vi "3-Midbrain.vi"() -> ()   [LabVIEW 2010]
doc: "This VI acts as the MIDbrain in the Olin Robotics Architecture. It interacts with neural clusters on both the Forebrain and Hindbrain as shown in teh respective control panel dynamic documentation diagrams."
uses:
  3-Midbrain/3.3-What/_typedefs/3.3-What Sensor Typedef.ctl
  3-Midbrain/3.3-What/_typedefs/3.3.1-LIDAR Data Typedef.ctl
  4-High Neurons/4.2-Where Sensor Typedef.ctl
  4-High Neurons/Current GPS Data.ctl
  3-Midbrain/3.2-Where/_typedefs/3.2.1-VectorNav Data.ctl
  4-High Neurons/4.4-How Sensor Typedef.ctl
  4-High Neurons/4.0-Midbrain State.ctl
  4-High Neurons/4.1.1-Act Joystick.ctl
  4-High Neurons/4.1-Act Control Typedef.ctl
  4-High Neurons/4.1.0-Datatype Typedef.ctl
  4-High Neurons/4.0-Super Heart Beat.ctl
  3-Midbrain/3.0-Global.vi
panel:
  out "4.0-Midbrain State 2":T1
  in  "Tabs!":T2(tab)
  out "XY Graph":cluster{i32[], "Speed By Path":dbl[]}[](graph)
  out "4.1.1-Joystick Data":T3 {"Right" scale=-32767.0..32767.0; "Left" scale=-32767.0..32767.0; "Yaw" scale=-32767.0..32767.0; "Roll" scale=-32767.0..32767.0; "Pitch" scale=-32767.0..32767.0}
  out "4.2-Where Am I? Sensor":T4 {"4.2.2- Current GPS Data"."Longitude (dd.mmmmmm)" format="%#.6g"; "4.2.2- Current GPS Data"."Lattitude (dd.mmmmmm)" format="%#.6g"}
  out "4.3-What's Around Me? Sensor":T7
  out "4.4-How Am I? Sensor":T9
  out "4.7-UDP Debug":T11
  in  "4.1 Act Control From GUI":T12
  out "Midbrain Heart Beat":bool
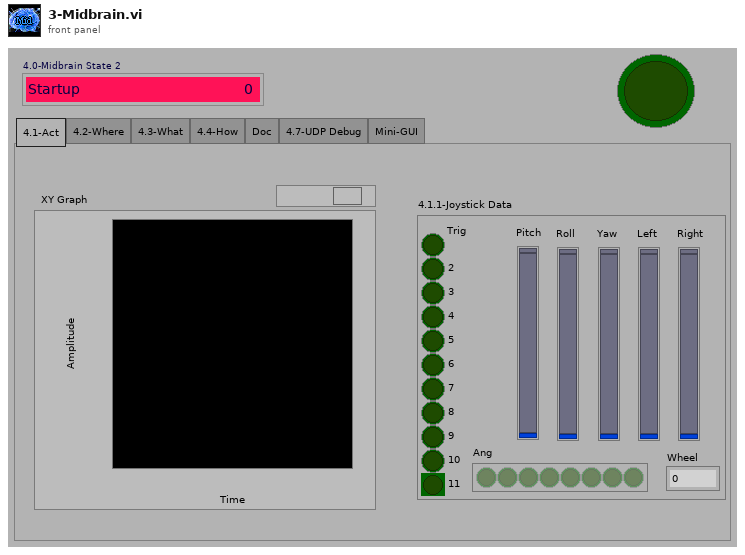
[diagram p1: front panel]
types:
  T1 = typedef "4.0-Midbrain State.ctl" = enum16{"Startup", "Waiting to Run", "Running-OlinOval", "Running-ChannelFollow", "Running-WallFollow", "Running-OpenTransit", "Running-Joystick Training", "Shutdown", "Restart", "New IP"}
  T2 = enum32{"4.1-Act", "4.2-Where", "4.3-What", "4.4-How", "Doc", "4.7-UDP Debug", "Mini-GUI"}
  T3 = typedef "4.1.1-Act Joystick.ctl" = cluster{"Trig":bool, "2":bool, "3":bool, "4":bool, "5":bool, "6":bool, "7":bool, "8":bool, "9":bool, "10":bool, "11":bool, "Pitch":i32, "Ang":bool[], "Wheel":dbl, "Roll":i32, "Yaw":i32, "Left":i32, "Right":i32}
  T4 = typedef "4.2-Where Sensor Typedef.ctl" = cluster{"4.2.2- Current GPS Data":T5, "4.2.1-VectorNav Data":T6, "4.2.1-VectorNav Status":string}
  T5 = typedef "Current GPS Data.ctl" = cluster{"Lattitude (dd.mmmmmm)":ext, "Longitude (dd.mmmmmm)":ext, "EST Time":timestamp}
  T6 = typedef "3.2.1-VectorNav Data.ctl" = cluster{"Yaw":dbl, "Pitch":dbl, "Roll":dbl}
  T7 = typedef "3.3-What Sensor Typedef.ctl" = cluster{"LIDAR Data":T8}
  T8 = typedef "3.3.1-LIDAR Data Typedef.ctl" = cluster{"Angle array":dbl[], "Magnitude array ":dbl[]}
  T9 = typedef "4.4-How Sensor Typedef.ctl" = cluster{"Motor Speed Integer":i32, "Drive Position Integer":i32, "Lidar Position Integer":i32, "Lidar Motor Position Integer":i32, "Steering Position Integer":i32, "Battery Voltage Fxp":dbl, "Drive Encoder Cable Check":bool, "Lidar Drive Encoder Cable Check":bool, "Steer Encoder Cable Check":bool, "Lidar Pos Encoder Cable Check":bool, "Mod Buttons & Blinky Cable Check":bool, "Lidar Data Cable Check":bool, "Drive Motor Cable Check":bool, "Vector Nav Cable Check":bool, "Lidar Drive Cable Check":bool, "Steer Drive Cable Check":bool, "Reverse?":bool, "2.1  Steering Control Voltage":dbl, "2.1 Drive Control Voltage":dbl, "2.1  Lidar Control Voltage":dbl, "2.5.7 A*B":dbl, "2.1  Steering PID Output":dbl, "2.1 Drive PID Output":dbl, "2.1  Lidar PID Output":dbl, "2.1.1 Drive Error":dbl, "2.1.1 Drive Error I":dbl, "2.1.1 Drive Error D":dbl, "2.1.2 Steering Error":dbl, "2.1.2 Steering Error I":dbl, "2.1.2 Steering Error D":dbl, "2.1.3 Lidar Error":dbl, "2.1.3 Lidar Error I":dbl, "2.1.3 Lidar Error D":dbl, "VectorNav Ack Query":bool, "VectorNav Read Byte":u8, "VectorNav Read Status":enum16{"Waiting", "Reading", "Done"}, "4.0-Midbrain State":T1}
  T10 = typedef "4.0-Super Heart Beat.ctl" = cluster{"Loop Period":u32, "HB":bool, "Last Ran":u32}
  T11 = cluster{"4.7.1-Act Super HB":T10, "4.7.2-Where Super HB":T10, "4.7.3-What Super HB":T10, "4.7.4-How Super HB":T10, "4.7.1-Act UDP Error":errorcluster, "4.7.2-Where UDP Error":errorcluster, "4.7.3-What UDP Error":errorcluster, "4.7.4-How UDP Error":errorcluster, "4.7-IP Address":string}
  T12 = typedef "4.1-Act Control Typedef.ctl" = cluster{"4.1.0 Data":variant, "Type of Data":T13, "E-Stop":bool, "Restart":bool, "New IP":bool, "Begin":bool, "Time":i32, "Shutdown":bool}
  T13 = typedef "4.1.0-Datatype Typedef.ctl" = enum16{"4.1.0-Empty Data", "4.1.1-Joystick Data", "4.1.2-Behavioral Data"}
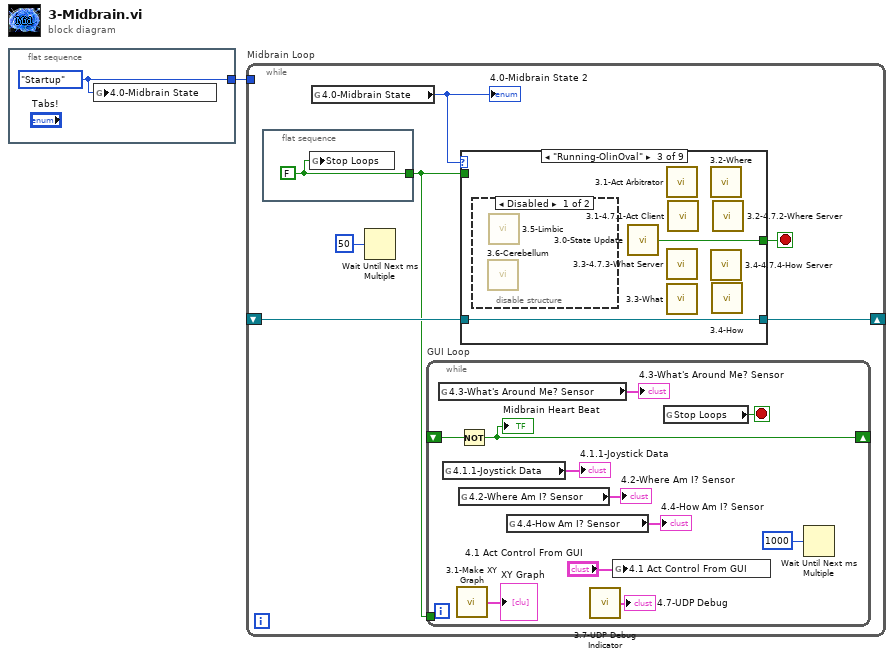
[diagram p0: block diagram]
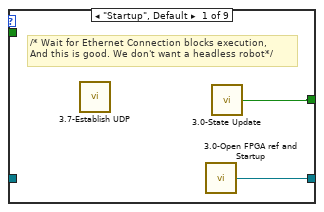
[diagram p2: hidden frame]
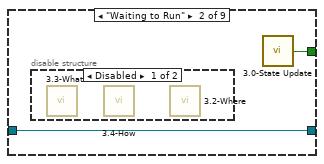
[diagram p3: hidden frame]
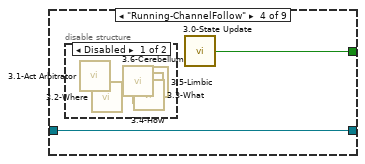
[diagram p6: hidden frame]
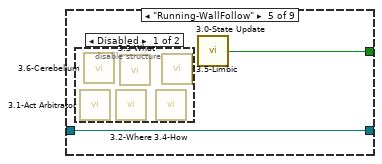
[diagram p8: hidden frame]
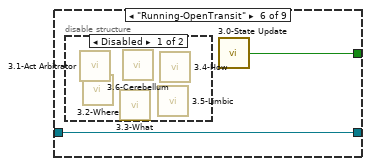
[diagram p10: hidden frame]
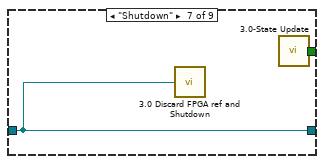
[diagram p12: hidden frame]
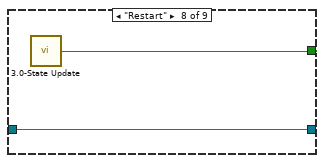
[diagram p13: hidden frame]
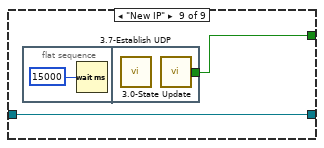
[diagram p14: hidden frame]
diagram:
  n1 = flat-sequence {
    tunnel: [w2] -> w1
    frame #0 {
      w2 = 4.0-Midbrain_State."Startup" ("4.0-Midbrain State")
      n2 = global write "3.0-Global.vi" "4.0-Midbrain State"(w2) -> ()
    }
  }
  n3 = while "Midbrain Loop" {
    shift-right: [w7] -> _
    shift-left: _ -> [w6]
    tunnel: w1 -> [_]
    stop <- w3 stop-if-true
    n4 = flat-sequence {
      tunnel: [w20] -> w4
      frame #0 {
        w20 = FALSE ("Flow Ctrl Stop")
        n5 = global write "3.0-Global.vi" "Stop Loops"(w20) -> ()
      }
    }
    n6 = global read "3.0-Global.vi" "4.0-Midbrain State"() -> (w8:T1)
    "4.0-Midbrain State 2" <- w8
    n7 = Wait Until Next ms Multiple(millisecond multiple=u32 50) -> ()  [unwired: 1 out]
    n8 = while "GUI Loop" {
      shift-right: [w10] -> _
      shift-left: _ -> [w11]
      tunnel: w4 -> [_]
      stop <- w19 stop-if-true
      n9 = global read "3.0-Global.vi" "4.3-What's Around Me? Sensor"() -> (→"4.3-What's Around Me? Sensor":T7)
      n10 = global read "3.0-Global.vi" "4.1.1-Joystick Data"() -> (→"4.1.1-Joystick Data":T3)
      n11 = call "3.1-Make XY Graph.vi"() -> ("Array"=→"XY Graph":cluster{i32[], "Speed By Path":dbl[]}[])
      n12 = Not(x=w11) -> (.not. x?=w10:bool)
      "Midbrain Heart Beat" <- w10
      n13 = global read "3.0-Global.vi" "4.2-Where Am I? Sensor"() -> (→"4.2-Where Am I? Sensor":T4)
      n14 = global read "3.0-Global.vi" "4.4-How Am I? Sensor"() -> (→"4.4-How Am I? Sensor":T9)
      n15 = call "3.7-UDP Debug Indicator.vi"() -> ("4.7-UDP Debug"=→"4.7-UDP Debug":T11)
      n16 = global write "3.0-Global.vi" "4.1 Act Control From GUI"("4.1 Act Control From GUI") -> ()
      n17 = global read "3.0-Global.vi" "Stop Loops"() -> (w19:bool)
      n18 = Wait Until Next ms Multiple(millisecond multiple=u32 1000) -> ()  [unwired: 1 out]
    }
    n19 = case shown="\"Running-OlinOval\"" w8 {
      tunnel: [w22 w24 w26 w28 w30 w32 w34 w36 w38] -> w7
      tunnel: w6 -> [_ w24 w26 w28 w30 w32 w34 w36 w38]
      tunnel: w4 -> [_ _ _ _ _ _ _ _ _]
      tunnel: [w21 w23 w25 w27 w29 w31 w33 w35 w37] -> w3
      frame "Startup", Default {
        # "/* Wait for Ethernet Connection blocks execution,\nAnd this is good. We don't want a headless robot*/"
        n20 = call "3.7-Establish UDP.vi"() -> ()  [unwired: 12 in]
        n21 = call "3.0-Open FPGA ref and Startup.vi"() -> ("queue out"=w22:refnum<queue>)
        n22 = call "3.0-State Update.vi"() -> ("End Program"=w21:bool)  [unwired: 1 in]
      }
      frame "Waiting to Run" {
        n23 = disable-structure shown="Disabled" {
          frame Disabled {
            n24 = call "3.3-What.vi"() -> ()  [unwired: 2 in, 1 out]
            n25 = call "3.4-How.vi"() -> ()  [unwired: 1 in]
            n26 = call "3.2-Where.vi"() -> ()  [unwired: 1 in]
          }
          frame Enabled {
          }
        }
        n27 = call "3.0-State Update.vi"() -> ("End Program"=w23:bool)  [unwired: 1 in]
      }
      frame "Running-OlinOval" {
        n28 = disable-structure shown="Disabled" {
          frame Disabled {
            n29 = call "3.6-Cerebellum.vi"() -> ()  [unwired: 12 in]
            n30 = call "3.5-Limbic.vi"() -> ()  [unwired: 12 in]
          }
          frame Enabled {
          }
        }
        n31 = call "3.0-State Update.vi"() -> ("End Program"=w25:bool)  [unwired: 1 in]
        n32 = call "3.1-Act Arbitrator.vi"() -> ()  [unwired: 1 in]
        n33 = call "3.3-4.7.3-What Server.vi"() -> ()  [unwired: 12 in]
        n34 = call "3.3-What.vi"() -> ()  [unwired: 2 in, 1 out]
        n35 = call "3.1-4.7.1-Act Client.vi"() -> ()  [unwired: 12 in]
        n36 = call "3.2-Where.vi"() -> ()  [unwired: 1 in]
        n37 = call "3.4-4.7.4-How Server.vi"() -> ()  [unwired: 1 in]
        n38 = call "3.4-How.vi"() -> ()  [unwired: 1 in]
        n39 = call "3.2-4.7.2-Where Server.vi"() -> ()  [unwired: 12 in]
      }
      frame "Running-ChannelFollow" {
        n40 = disable-structure shown="Disabled" {
          frame Disabled {
            n41 = call "3.1-Act Arbitrator.vi"() -> ()  [unwired: 1 in]
            n42 = call "3.2-Where.vi"() -> ()  [unwired: 1 in]
            n43 = call "3.6-Cerebellum.vi"() -> ()  [unwired: 12 in]
            n44 = call "3.4-How.vi"() -> ()  [unwired: 1 in]
            n45 = call "3.3-What.vi"() -> ()  [unwired: 2 in, 1 out]
            n46 = call "3.5-Limbic.vi"() -> ()  [unwired: 12 in]
          }
          frame Enabled {
          }
        }
        n47 = call "3.0-State Update.vi"() -> ("End Program"=w27:bool)  [unwired: 1 in]
      }
      frame "Running-WallFollow" {
        n48 = disable-structure shown="Disabled" {
          frame Disabled {
            n49 = call "3.1-Act Arbitrator.vi"() -> ()  [unwired: 1 in]
            n50 = call "3.6-Cerebellum.vi"() -> ()  [unwired: 12 in]
            n51 = call "3.2-Where.vi"() -> ()  [unwired: 1 in]
            n52 = call "3.3-What.vi"() -> ()  [unwired: 2 in, 1 out]
            n53 = call "3.4-How.vi"() -> ()  [unwired: 1 in]
            n54 = call "3.5-Limbic.vi"() -> ()  [unwired: 12 in]
          }
          frame Enabled {
          }
        }
        n55 = call "3.0-State Update.vi"() -> ("End Program"=w29:bool)  [unwired: 1 in]
      }
      frame "Running-OpenTransit" {
        n56 = disable-structure shown="Disabled" {
          frame Disabled {
            n57 = call "3.1-Act Arbitrator.vi"() -> ()  [unwired: 1 in]
            n58 = call "3.2-Where.vi"() -> ()  [unwired: 1 in]
            n59 = call "3.3-What.vi"() -> ()  [unwired: 2 in, 1 out]
            n60 = call "3.6-Cerebellum.vi"() -> ()  [unwired: 12 in]
            n61 = call "3.5-Limbic.vi"() -> ()  [unwired: 12 in]
            n62 = call "3.4-How.vi"() -> ()  [unwired: 1 in]
          }
          frame Enabled {
          }
        }
        n63 = call "3.0-State Update.vi"() -> ("End Program"=w31:bool)  [unwired: 1 in]
      }
      frame "Shutdown" {
        n64 = call "3.0 Discard FPGA ref and Shutdown.vi"("queue out"=w34) -> ()
        n65 = call "3.0-State Update.vi"() -> ("End Program"=w33:bool)  [unwired: 1 in]
      }
      frame "Restart" {
        n66 = call "3.0-State Update.vi"() -> ("End Program"=w35:bool)  [unwired: 1 in]
      }
      frame "New IP" {
        n67 = flat-sequence {
          tunnel: [w40] -> w37
          frame #0 {
            n68 = Wait (ms)(milliseconds to wait=u32 15000) -> ()  [unwired: 1 out]
          }
          frame #1 {
            n69 = call "3.7-Establish UDP.vi"() -> ()  [unwired: 12 in]
            n70 = call "3.0-State Update.vi"() -> ("End Program"=w40:bool)  [unwired: 1 in]
          }
        }
      }
    }
  }
